vi "Build System Param Arrays.vi"(8 "Error In":errorcluster, 11 "Input String Array":string[](array[string])) -> (0 "Error Out":errorcluster, 3 "Output String Array":string[](array[string]))   [LabVIEW 2017]
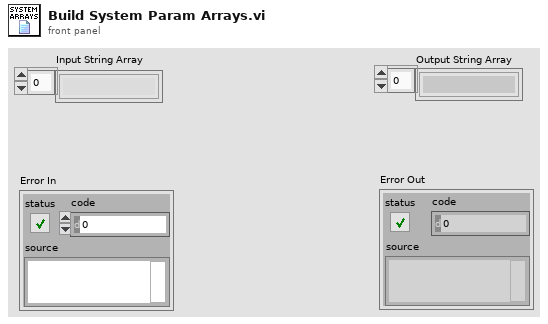
[diagram p1: front panel]
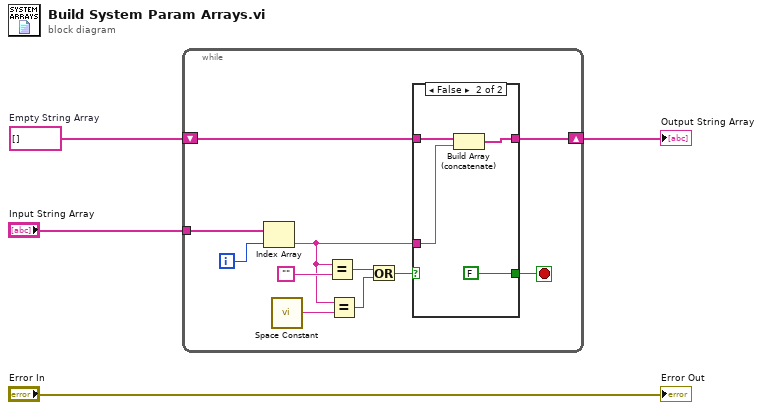
[diagram p0: block diagram]
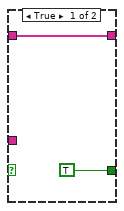
[diagram p2: hidden frame]
diagram:
  w4 = string[] []  # Empty String Array
  n1 = while {
    shift-right: [w6] -> w3
    shift-left: w4 -> [w7]
    tunnel: "Input String Array" -> [w15]
    i -> [w14]
    stop <- w8 stop-if-true
    n2 = Index Array(array=w15, index=w14) -> (element=w5:string)
    n3 = call <vilib>:"Space Constant.vi"() -> ("String"=w12:string)
    n4 = Equal?(x=w5, y="") -> (x = y?=w10:bool)
    n5 = Equal?(x=w5, y=w12) -> (x = y?=w9:bool)
    n6 = Or(x=w10, y=w9) -> (x .or. y?=w11:bool)
    n7 = case shown="False" w11 {
      tunnel: [TRUE FALSE] -> w8
      tunnel: w7 -> [w16 w20]
      tunnel: [w16 w18] -> w6
      tunnel: w5 -> [_ w19]
      frame True {
      }
      frame False {
        n8 = Build Array (concatenate)(w20, w19) -> (w18:string[])
      }
    }
  }
  "Output String Array" <- w3
  "Error Out" <- "Error In"
